vi "总磷总氮启动参数对话框.vi"() -> (2 "确认":bool, 3 "元素":cluster{"命令":string, "data":variant})   [LabVIEW 2016, in "斯坦道氨氮.lvlib"]
panel:
  in  "协议":u16(ring)=2 items=["斯坦道协议"=1, "国标协议"=2]
  in  "维护模式":bool=TRUE
  out "标液值":dbl caption="标液值："
  in  "取消":bool
  in  "确定":bool
  in  "量程切换":u16(ring)=2 items=["高量程", "低量程", "自动"]
  in  "站号":u16(ring)=1 items=["总氮"=2, "总磷"=1, "磷酸盐"=4]
  in  "控制命令":T1(ring)
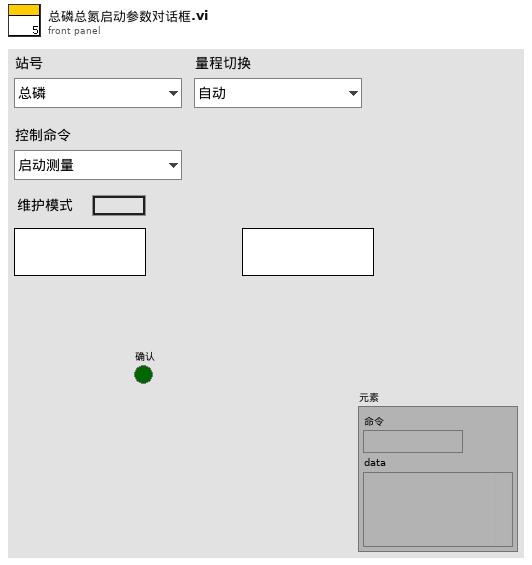
[diagram p1: front panel]
types:
  T1 = enum16{"启动测量", "标样核查", "零点核查", "跨度核查", "空白测试", "平行样测试", "加标回收", "空白校准", "标样校准", "初始化（清洗）", "停止测试", "仪器重启", "校时", "模式设置", "测量间隔设置"}
  T2 = typedef "LVStringsAndValuesArrayTypeDef_U16.ctl" = cluster{"String":string, "Value":u16}[]
  T3 = typedef "操作日志字段定义.ctl" = cluster{"时间":timestamp, "参数":string, "日志信息":string, "流程参数":string}
  T4 = cluster{"站号":u16, "量程切换":enum32{"H", "L", "AUTO"}, "控制命令":enum16{"启动测量", "标样核查", "零点核查", "跨度核查", "空白测试", "平行样测试", "加标回收", "空白校准", "标样校准", "初始化（清洗）", "停止测试", "仪器重启", "校时", "模式设置", "测量间隔设置", "盲样测试"}, "模式设置":enum16{"待机", "连续模式", "周期模式", "定点模式", "受控模式", "手动模式"}, "测量间隔":u16}
  T5 = cluster{"总磷跨度值":dbl, "总磷零点标准液浓度":dbl, "总磷跨度标准液浓度":dbl, "总磷标准液标准浓度":dbl, "总氮跨度值":dbl, "总氮零点标准液浓度":dbl, "总氮跨度标准液浓度":dbl, "总氮标准液标准浓度":dbl, "COD跨度值":dbl, "COD零点标准液浓度":dbl, "COD跨度标准液浓度":dbl, "COD标准液标准浓度":dbl, "氨氮跨度值":dbl, "氨氮零点标准液浓度":dbl, "氨氮跨度标准液浓度":dbl, "氨氮标准液标准浓度":dbl, "磷酸盐跨度值":dbl, "磷酸盐零点标准液浓度":dbl, "磷酸盐跨度标准液浓度":dbl, "磷酸盐标准液标准浓度":dbl, "硝氮跨度值":dbl, "硝氮零点标准液浓度":dbl, "硝氮跨度标准液浓度":dbl, "硝氮标准液标准浓度":dbl, "亚硝氮跨度值":dbl, "亚硝氮零点标准液浓度":dbl, "亚硝氮跨度标准液浓度":dbl, "亚硝氮标准液标准浓度":dbl, "硫化物跨度值":dbl, "硫化物零点标准液浓度":dbl, "硫化物跨度标准液浓度":dbl, "硫化物标准液标准浓度":dbl, "硅酸盐跨度值":dbl, "硅酸盐零点标准液浓度":dbl, "硅酸盐跨度标准液浓度":dbl, "硅酸盐标准液标准浓度":dbl, "总磷零点标准液偏差":dbl, "总磷跨度标准液偏差":dbl, "总磷标准液标准偏差":dbl, "总氮零点标准液偏差":dbl, "总氮跨度标准液偏差":dbl, "总氮标准液标准偏差":dbl, "COD零点标准液偏差":dbl, "COD跨度标准液偏差":dbl, "COD标准液标准偏差":dbl, "氨氮零点标准液偏差":dbl, "氨氮跨度标准液偏差":dbl, "氨氮标准液标准偏差":dbl, "磷酸盐零点标准液偏差":dbl, "磷酸盐跨度标准液偏差":dbl, "磷酸盐标准液标准偏差":dbl, "硝氮零点标准液偏差":dbl, "硝氮跨度标准液偏差":dbl, "硝氮标准液标准偏差":dbl, "亚硝氮零点标准液偏差":dbl, "亚硝氮跨度标准液偏差":dbl, "亚硝氮标准液标准偏差":dbl, "硫化物零点标准液偏差":dbl, "硫化物跨度标准液偏差":dbl, "硫化物标准液标准偏差":dbl, "硅酸盐零点标准液偏差":dbl, "硅酸盐跨度标准液偏差":dbl, "硅酸盐标准液标准偏差":dbl, "氟化物跨度值":dbl, "氟化物零点标准液浓度":dbl, "氟化物跨度标准液浓度":dbl, "氟化物标准液标准浓度":dbl, "氟化物零点标准液偏差":dbl, "氟化物跨度标准液偏差":dbl, "氟化物标准液标准偏差":dbl, "CODMn跨度值":dbl, "CODMn零点标准液浓度":dbl, "CODMn跨度标准液浓度":dbl, "CODMn标准液标准浓度":dbl, "CODMn零点标准液偏差":dbl, "CODMn跨度标准液偏差":dbl, "CODMn标准液标准偏差":dbl}
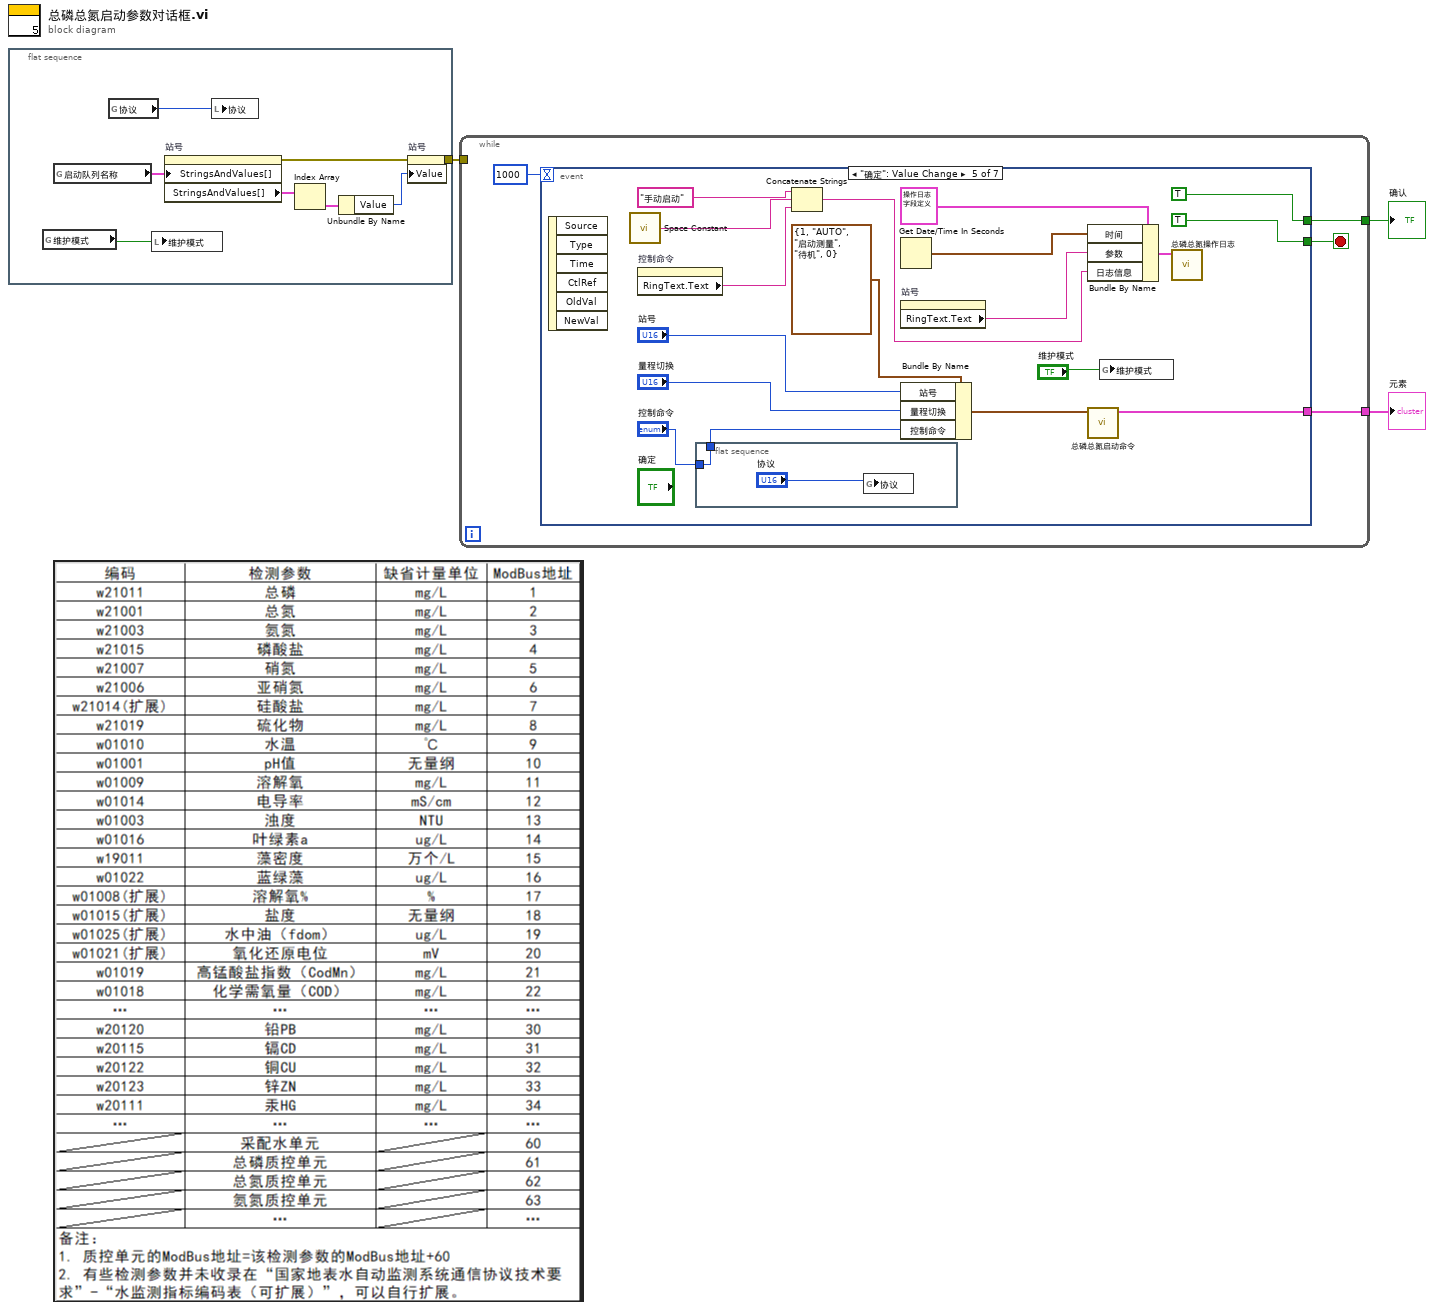
[diagram p0: block diagram]
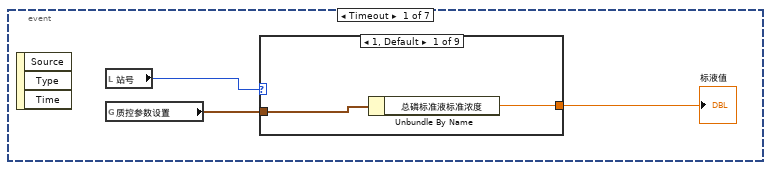
[diagram p2: hidden frame]
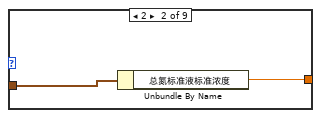
[diagram p3: hidden frame]
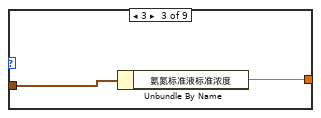
[diagram p4: hidden frame]
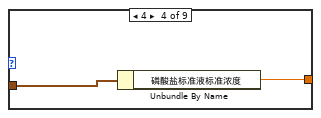
[diagram p5: hidden frame]
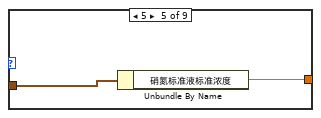
[diagram p6: hidden frame]
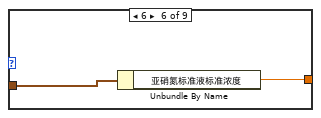
[diagram p7: hidden frame]
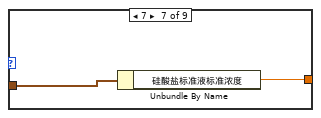
[diagram p8: hidden frame]
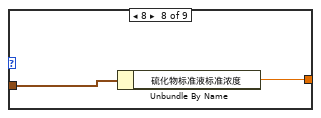
[diagram p9: hidden frame]
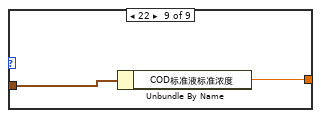
[diagram p10: hidden frame]
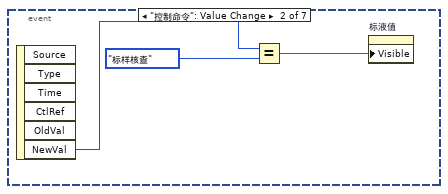
[diagram p11: hidden frame]
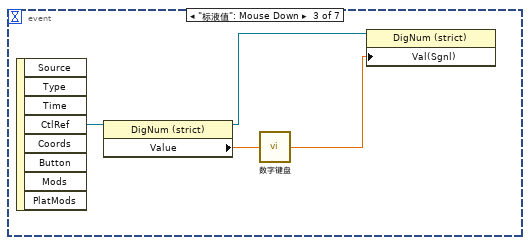
[diagram p12: hidden frame]
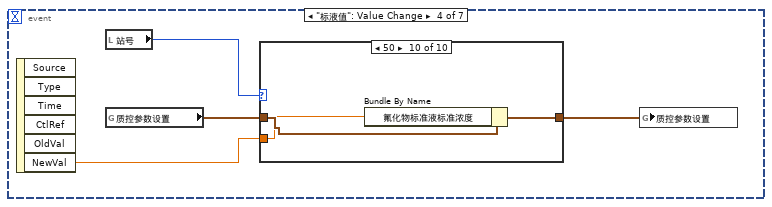
[diagram p13: hidden frame]
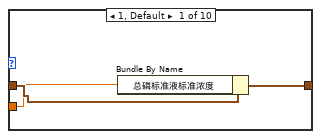
[diagram p14: hidden frame]
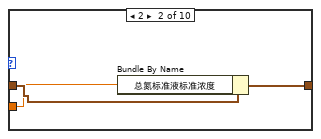
[diagram p15: hidden frame]
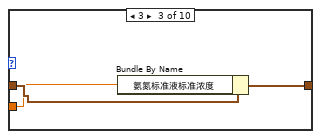
[diagram p16: hidden frame]
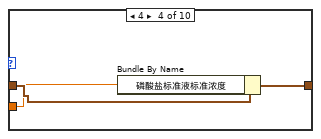
[diagram p17: hidden frame]
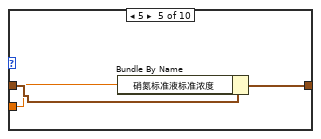
[diagram p18: hidden frame]
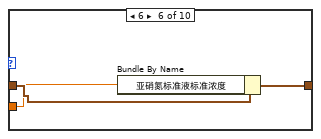
[diagram p19: hidden frame]
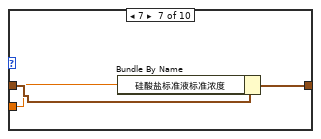
[diagram p20: hidden frame]
diagram:
  n1 = flat-sequence {
    tunnel: [w6] -> w1
    frame #0 {
      n2 = global read "VAR总磷总氮全局变量.vi" "维护模式"() -> (w5:bool)
      n3 = global read "model config var.vi" "启动队列名称"() -> (w11:cluster{"String":string, "Value":u16}[])
      n4 = global read "总磷总氮断电保存全局变量.vi" "协议"() -> (w4:u16)
      n5 = local write "维护模式"(w5) -> ()
      n6 = property on="站号" class="Ring (strict)"("StringsAndValues[]"=w11) -> (error out=w10:errorcluster, "StringsAndValues[]"=w9:T2)  [unwired: 2 in, 1 out]
      n7 = local write "协议"(w4) -> ()
      n8 = Index Array(array=w9) -> (element=w8:cluster{"String":string, "Value":u16})  [unwired: 1 in]
      n9 = Unbundle By Name(w8) -> ("Value"=w7:u16)
      n10 = property on="站号" class="Ring (strict)"(error in=w10, "Value"=w7) -> (error out=w6:errorcluster)  [unwired: 1 in, 1 out]
    }
  }
  n11 = while {
    tunnel: [w13] -> w3
    tunnel: [w12] -> w2
    tunnel: w1 -> [_]
    stop <- w15 stop-if-true
    n12 = event shown="[4] \"确定\": Value Change" {
      selector: _ -> [_ _ _ _ _ _ _]
      dyn-events: _ -> [_ _ _ _ _ _ _]
      timeout: 1000 -> [_ _ _ _ _ _ _]
      tunnel: [_ _ _ _ TRUE _ TRUE] -> w15
      tunnel: [_ _ _ _ TRUE _ _] -> w13
      tunnel: [_ _ _ _ w93 _ _] -> w12
      event Timeout {
        n13 = event-data() -> ()  [unwired: 1 in, 3 out]
        n14 = local read "站号"() -> (w17:u16)
        n15 = global read "总磷总氮断电保存全局变量.vi" "质控参数设置"() -> (w18:T5)
        n16 = case shown="1, Default" w17 {
          tunnel: w18 -> [w20 w22 w24 w26 w28 w30 w32 w34 w36]
          tunnel: [w19 w21 w23 w25 w27 w29 w31 w33 w35] -> w16
          frame 1, Default {
            n17 = Unbundle By Name(w20) -> ("总磷标准液标准浓度"=w19:dbl)
          }
          frame 2 {
            n18 = Unbundle By Name(w22) -> ("总氮标准液标准浓度"=w21:dbl)
          }
          frame 3 {
            n19 = Unbundle By Name(w24) -> ("氨氮标准液标准浓度"=w23:dbl)
          }
          frame 4 {
            n20 = Unbundle By Name(w26) -> ("磷酸盐标准液标准浓度"=w25:dbl)
          }
          frame 5 {
            n21 = Unbundle By Name(w28) -> ("硝氮标准液标准浓度"=w27:dbl)
          }
          frame 6 {
            n22 = Unbundle By Name(w30) -> ("亚硝氮标准液标准浓度"=w29:dbl)
          }
          frame 7 {
            n23 = Unbundle By Name(w32) -> ("硅酸盐标准液标准浓度"=w31:dbl)
          }
          frame 8 {
            n24 = Unbundle By Name(w34) -> ("硫化物标准液标准浓度"=w33:dbl)
          }
          frame 22 {
            n25 = Unbundle By Name(w36) -> ("COD标准液标准浓度"=w35:dbl)
          }
        }
        "标液值" <- w16
      }
      event "控制命令": Value Change {
        n26 = event-data() -> ("NewVal"=w39:T1)  [unwired: 1 in, 5 out]
        n27 = Equal?(x=w39, y=T1."标样核查") -> (x = y?=w37:bool)
        n28 = property on="标液值" class="DigNum (strict)"("Visible"=w37) -> ()  [unwired: 2 in, 2 out]
      }
      event "标液值": Mouse Down {
        n29 = event-data() -> ("CtlRef"=w43:refnum<vi>)  [unwired: 1 in, 7 out]
        n30 = property class="DigNum (strict)"(reference=w43) -> (reference out=w40:refnum<vi>, "Value"=w42:dbl)  [unwired: 1 in, 1 out]
        n31 = call "数字键盘.vi"("OldNumber"=w42) -> ("NewNumber"=w41:dbl)
        n32 = property class="DigNum (strict)"(reference=w40, "Val(Sgnl)"=w41) -> ()  [unwired: 1 in, 2 out]
      }
      event "标液值": Value Change {
        n33 = event-data() -> ("NewVal"=w45:dbl)  [unwired: 1 in, 5 out]
        n34 = local read "站号"() -> (w47:u16)
        n35 = global read "总磷总氮断电保存全局变量.vi" "质控参数设置"() -> (w46:T5)
        n36 = case shown="50" w47 {
          tunnel: w46 -> [w50 w53 w56 w59 w62 w65 w68 w71 w74 w77]
          tunnel: [w48 w51 w54 w57 w60 w63 w66 w69 w72 w75] -> w44
          tunnel: w45 -> [w49 w52 w55 w58 w61 w64 w67 w70 w73 w76]
          frame 1, Default {
            n37 = Bundle By Name(cluster=w50, "总磷标准液标准浓度"=w49) -> (w48:T5)
          }
          frame 2 {
            n38 = Bundle By Name(cluster=w53, "总氮标准液标准浓度"=w52) -> (w51:T5)
          }
          frame 3 {
            n39 = Bundle By Name(cluster=w56, "氨氮标准液标准浓度"=w55) -> (w54:T5)
          }
          frame 4 {
            n40 = Bundle By Name(cluster=w59, "磷酸盐标准液标准浓度"=w58) -> (w57:T5)
          }
          frame 5 {
            n41 = Bundle By Name(cluster=w62, "硝氮标准液标准浓度"=w61) -> (w60:T5)
          }
          frame 6 {
            n42 = Bundle By Name(cluster=w65, "亚硝氮标准液标准浓度"=w64) -> (w63:T5)
          }
          frame 7 {
            n43 = Bundle By Name(cluster=w68, "硅酸盐标准液标准浓度"=w67) -> (w66:T5)
          }
          frame 8 {
            n44 = Bundle By Name(cluster=w71, "硫化物标准液标准浓度"=w70) -> (w69:T5)
          }
          frame 22 {
            n45 = Bundle By Name(cluster=w74, "COD标准液标准浓度"=w73) -> (w72:T5)
          }
          frame 50 {
            n46 = Bundle By Name(cluster=w77, "氟化物标准液标准浓度"=w76) -> (w75:T5)
          }
        }
        n47 = global write "总磷总氮断电保存全局变量.vi" "质控参数设置"(w44) -> ()
      }
      event "确定": Value Change {
        n48 = event-data() -> ()  [unwired: 1 in, 6 out]
        n49 = call <vilib>:"Space Constant.vi"() -> ("String"=w84:string)
        n50 = property on="控制命令" class="Enum (strict)"() -> ("RingText.Text"=w85:string)  [unwired: 2 in, 2 out]
        n51 = flat-sequence {
          tunnel: "控制命令" -> [w97]
          tunnel: [w97] -> w78
          frame #0 {
            n52 = global write "总磷总氮断电保存全局变量.vi" "协议"("协议") -> ()
          }
        }
        n53 = Concatenate Strings("手动启动" ("日志信息"), w84, w85) -> (w81:string)
        n54 = Get Date/Time In Seconds() -> (seconds since 1Jan1904=w86:timestamp)
        n55 = property on="站号" class="Ring (strict)"() -> ("RingText.Text"=w83:string)  [unwired: 2 in, 2 out]
        n56 = Bundle By Name(cluster=T4 {"站号"=1, "量程切换"=enum."AUTO", "控制命令"=enum."启动测量", "模式设置"=enum."待机", "测量间隔"=0} ("参数"), "站号"="站号", "量程切换"="量程切换", "控制命令"=w78) -> (w91:T4)
        n57 = Bundle By Name(cluster=T3 {"时间"=timestamp(0 s since 1904-01-01), "参数"="", "日志信息"="", "流程参数"=""} ("data in"), "时间"=w86, "参数"=w83, "日志信息"=w81) -> (w87:T3)
        n58 = call "总磷总氮启动命令.vi"("参数"=w91) -> ("启动命令"=w93:cluster{"命令":string, "data":variant})  [unwired: 10 in]
        n59 = global write "VAR总磷总氮全局变量.vi" "维护模式"("维护模式") -> ()
        n60 = call "总磷总氮操作日志.vi"("data in"=w87) -> ()  [unwired: 10 in, 1 out]
      }
      event "协议": Value Change {
        n61 = event-data() -> ("NewVal"=w98:u16)  [unwired: 1 in, 5 out]
        n62 = global write "总磷总氮断电保存全局变量.vi" "协议"(w98) -> ()
      }
      event "取消": Value Change; Panel Close {
        n63 = event-data() -> ()  [unwired: 1 in, 3 out]
      }
    }
  }
  "元素" <- w2
  "确认" <- w3
